vi "Write Rotation.vi"(8 "error in (no error)":errorcluster, 10 "Rotation":enum16{"Clockwise", "CounterClockwise"}(ring), 11 "Cricket in":refnum<class "Cricket.lvclass">) -> (0 "error out":errorcluster, 3 "Cricket out":refnum<class "Cricket.lvclass">)   [LabVIEW 2021, in "Cricket.lvclass"]
uses:
  Cricket.lvclass
  Cricket.lvclass/Cricket.ctl
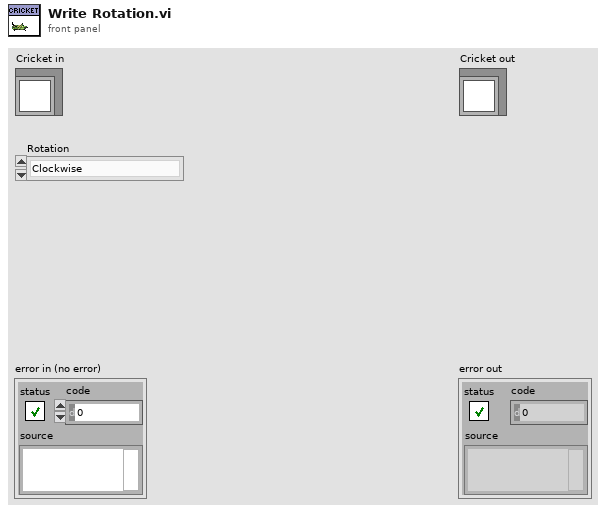
[diagram p1: front panel]
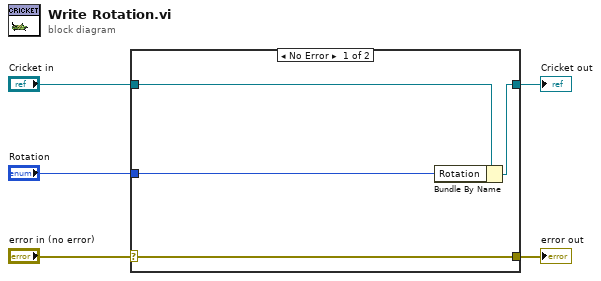
[diagram p0: block diagram]
diagram:
  n1 = case shown="No Error" "error in (no error)" {
    selector: "error in (no error)" -> [w9 w10]
    tunnel: [w9 w10] -> w4
    tunnel: [w7 w11] -> w2
    tunnel: "Cricket in" -> [w8 w11]
    tunnel: "Rotation" -> [w6 _]
    frame No Error {
      n2 = Bundle By Name(cluster=w8, "Rotation"=w6) -> (w7:refnum<class "Cricket.lvclass">)
    }
    frame Error {
    }
  }
  "error out" <- w4
  "Cricket out" <- w2
